vi "IsImplemented.vi"(4 "error in (no error)":errorcluster, 5 "strName":string, 6 "Read Data":bool, 7 "nInputHandle":u64) -> (0 "error out":errorcluster, 1 "GX_STATUS":i32, 2 "Result":bool=TRUE, 3 "nOutputHandle":u64)   [LabVIEW 2016, in "GxLVLib.lvlib"]
uses:
  GxLVLib.lvlib
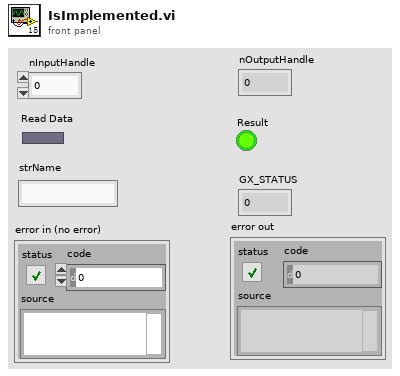
[diagram p1: front panel]
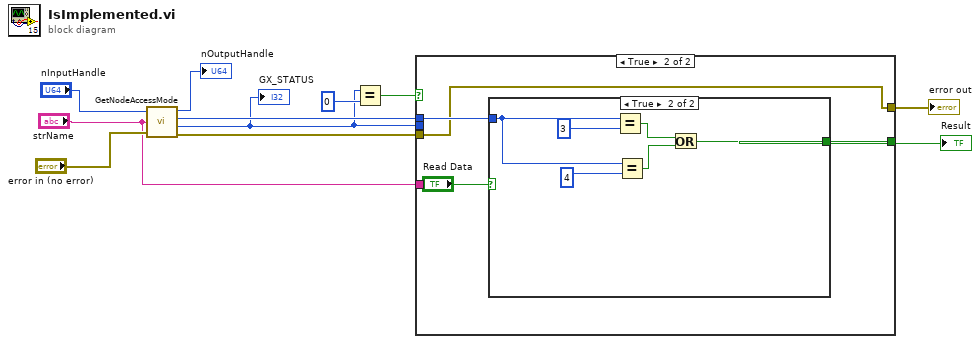
[diagram p0: block diagram]
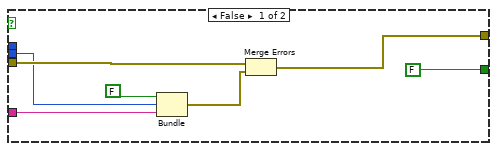
[diagram p2: hidden frame]
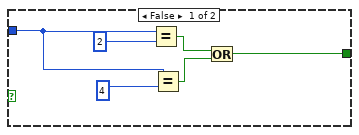
[diagram p3: hidden frame]
diagram:
  n1 = call "GetNodeAccessMode.vi"("nInputHandle"="nInputHandle", "strName"="strName", "error in (no error)"="error in (no error)") -> ("nOuputHandle"=→"nOutputHandle":u64, "pemAccessMode"=w6:i32, "GX_STATUS"=w3:i32, "error out"=w4:errorcluster)
  "GX_STATUS" <- w3
  n2 = Equal?(x=w3, y=0) -> (x = y?=w8:bool)
  n3 = case shown="True" w8 {
    tunnel: [FALSE w20] -> w7
    tunnel: w6 -> [_ w21]
    tunnel: w4 -> [w16 w19]
    tunnel: w3 -> [w14 _]
    tunnel: "strName" -> [w13 _]
    tunnel: [w12 w19] -> w1
    frame False {
      n4 = Bundle(FALSE, "GX_STATUS"=w14, "strName"=w13) -> (w17:cluster{bool, "GX_STATUS":i32, "strName":string})  [unwired: 1 in]
      n5 = Merge Errors(w16, w17) -> (w12:errorcluster)
    }
    frame True {
      n6 = case shown="True" "Read Data" {
        tunnel: w21 -> [w24 w30]
        tunnel: [w23 w32] -> w20
        frame False {
          n7 = Equal?(x=w24, y=2) -> (x = y?=w25:bool)
          n8 = Equal?(x=w24, y=4) -> (x = y?=w27:bool)
          n9 = Or(x=w25, y=w27) -> (x .or. y?=w23:bool)
        }
        frame True {
          n10 = Equal?(x=w30, y=3) -> (x = y?=w29:bool)
          n11 = Equal?(x=w30, y=4) -> (x = y?=w33:bool)
          n12 = Or(x=w29, y=w33) -> (x .or. y?=w32:bool)
        }
      }
    }
  }
  "error out" <- w1
  "Result" <- w7
